vi "Gen - Close VI.vi"(8 "Error In":errorcluster, 10 "Force Close? (F)":bool, 11 "Ref VI":refnum<vi>) -> (0 "Error Out":errorcluster)   [LabVIEW 2020]
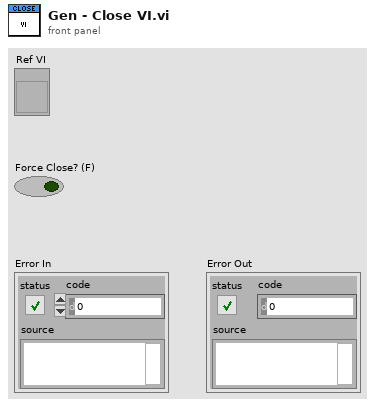
[diagram p1: front panel]
types:
  T1 = enum32{"invalid app kind", "Development System", "Run Time System", "Student Edition", "Embedded LabVIEW", "Evaluation", "Custom"}
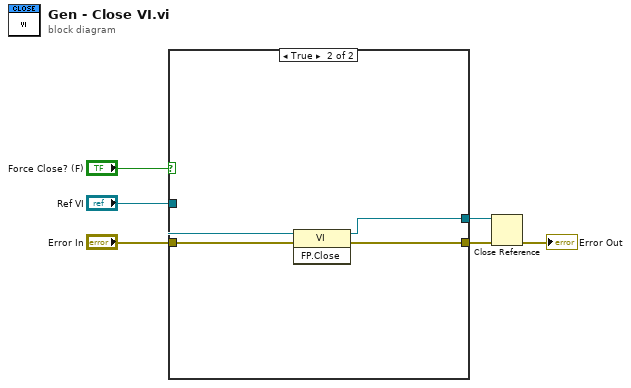
[diagram p0: block diagram]
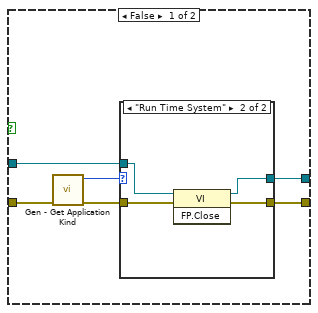
[diagram p2: hidden frame]
diagram:
  n1 = case shown="True" "Force Close? (F)" {
    tunnel: "Error In" -> [w11 w22]
    tunnel: [w12 w21] -> w5
    tunnel: "Ref VI" -> [w9 w19]
    tunnel: [w8 w20] -> w1
    frame False {
      n2 = call "Gen - Get Application Kind.vi"("Error In"=w11) -> ("Error Out"=w10:errorcluster, "Application:Kind"=w7:T1)  [unwired: 9 in]
      n3 = case shown="\"Run Time System\"" w7 {
        tunnel: [w14 w17] -> w12
        tunnel: w10 -> [w14 w18]
        tunnel: w9 -> [w13 w16]
        tunnel: [w13 w15] -> w8
        frame "invalid app kind", Default {
        }
        frame "Run Time System" {
          n4 = invoke class="VI" method="FP.Close"(reference=w16, error in=w18) -> (reference out=w15:refnum<vi>, error out=w17:errorcluster)  [unwired: 1 in, 1 out]
        }
      }
    }
    frame True {
      n5 = invoke class="VI" method="FP.Close"(reference=w19, error in=w22) -> (reference out=w20:refnum<vi>, error out=w21:errorcluster)  [unwired: 1 in, 1 out]
    }
  }
  n6 = Close Reference(reference=w1, error in (no error)=w5) -> (error out=→"Error Out":errorcluster)
